vi "SaveOneImage.vi"(7 "Save images path":path, 9 "XYZ stage coordinates of image":dbl[](array[numeric]), 10 "Image Number":i32, 11 "Image":T1(plugin-control)) -> ()   [LabVIEW 2016]
panel:
  in  "error in (no error)":errorcluster
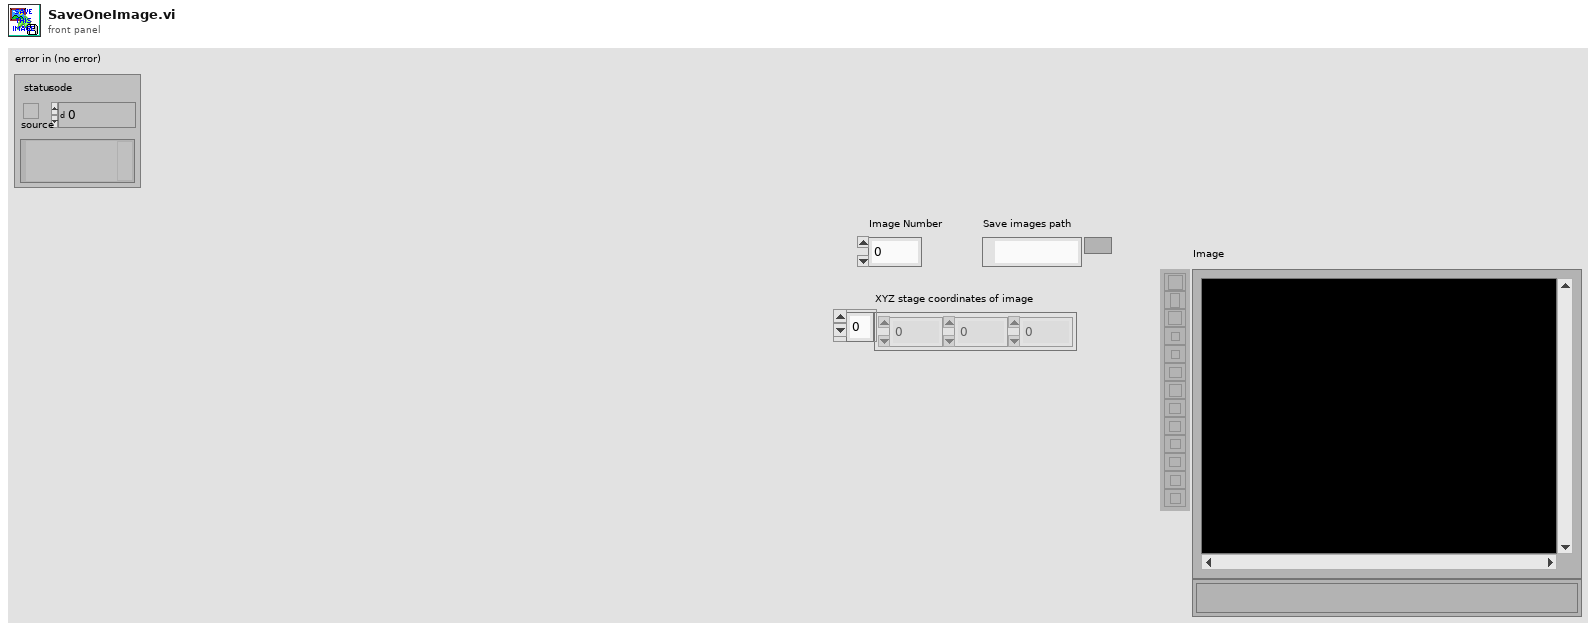
[diagram p1: front panel]
types:
  T1 = typedef "IMAQ Image.ctl" = refnum<image>
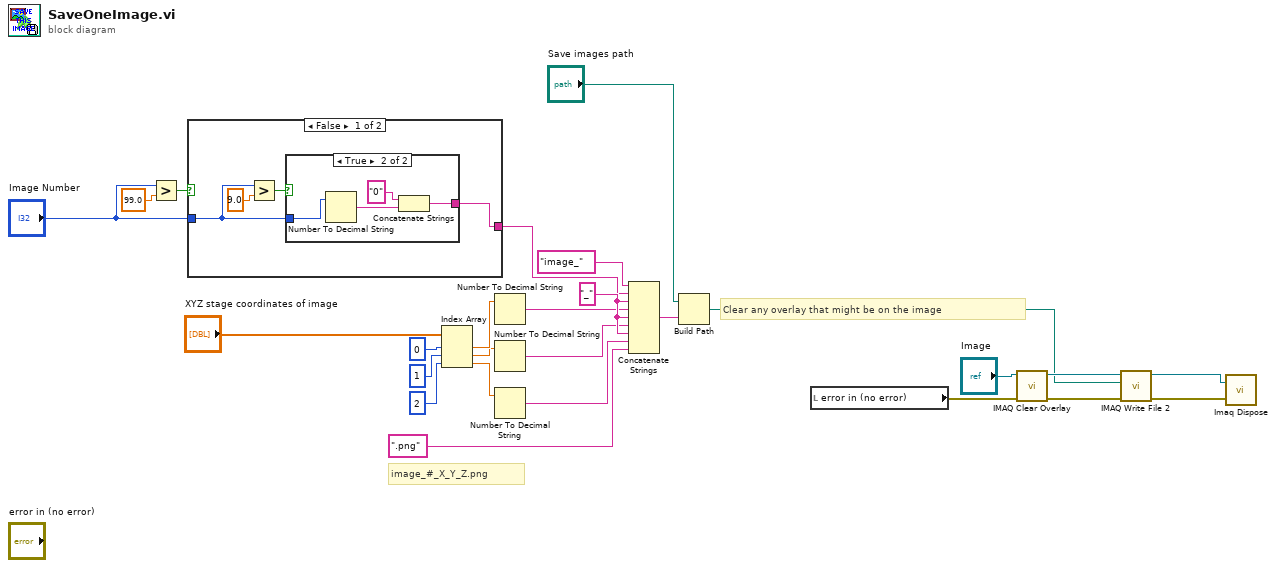
[diagram p0: block diagram]
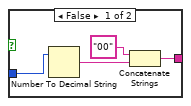
[diagram p2: hidden frame]
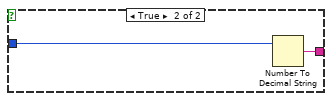
[diagram p3: hidden frame]
diagram:
  w17 = "_" ("string")
  # "image_#_X_Y_Z.png"
  # "Clear any overlay that might be on the image"
  n1 = Greater?(x="Image Number", y=99.0) -> (0:w12:bool)
  n2 = case shown="False" w12 {
    tunnel: "Image Number" -> [w27 w40]
    tunnel: [w29 w39] -> w16
    frame False {
      n3 = Greater?(x=w27, y=9.0) -> (0:w28:bool)
      n4 = case shown="True" w28 {
        tunnel: [w32 w35] -> w29
        tunnel: w27 -> [w31 w36]
        frame False {
          n5 = Number To Decimal String(number=w31) -> (decimal integer string=w34:string)  [unwired: 1 in]
          n6 = Concatenate Strings("00" ("string"), w34) -> (w32:string)
        }
        frame True {
          n7 = Number To Decimal String(number=w36) -> (decimal integer string=w38:string)  [unwired: 1 in]
          n8 = Concatenate Strings("0" ("string"), w38) -> (w35:string)
        }
      }
    }
    frame True {
      n9 = Number To Decimal String(number=w40) -> (decimal integer string=w39:string)  [unwired: 1 in]
    }
  }
  n10 = Index Array(array="XYZ stage coordinates of image", index #1=0 ("disabled index (col)"), index #2=1 ("disabled index (col)"), index #3=2 ("index (col)")) -> (element #1=w6:dbl, element #2=w2:dbl, element #3=w1:dbl)
  n11 = Number To Decimal String(number=w6) -> (decimal integer string=w15:string)  [unwired: 1 in]
  n12 = Number To Decimal String(number=w2) -> (decimal integer string=w14:string)  [unwired: 1 in]
  n13 = Number To Decimal String(number=w1) -> (decimal integer string=w13:string)  [unwired: 1 in]
  n14 = Concatenate Strings("image_" ("string"), w16, w17, w15, w17, w14, w17, w13, ".png" ("string")) -> (w26:string)
  n15 = Build Path(base path="Save images path", name or relative path=w26) -> (appended path=w19:path)
  n16 = local read "error in (no error)"() -> (w22:errorcluster)
  n17 = call "IMAQ Clear Overlay"("error in (no error)"=w22, "Image"="Image") -> ("error out"=w21:errorcluster, "Image Out"=w20:T1)  [unwired: 8 in]
  n18 = call-poly "IMAQ Write File 2"("error in (no error)"=w21, "File Path"=w19, "Image"=w20) -> ("error out"=w23:errorcluster, "Image Out (duplicate)"=w24:T1)  [unwired: 7 in]
  n19 = call "Imaq Dispose"("Image"=w24, "error in (no error)"=w23) -> ()  [unwired: 4 in, 1 out]
